vi "Increment Waveform.vi"(8 "error in (no error)":errorcluster, 11 "Model in":refnum<class "Model.lvclass">) -> (0 "error out":errorcluster, 3 "Model out":refnum<class "Model.lvclass">)   [LabVIEW 2016]
uses:
  Model.lvclass
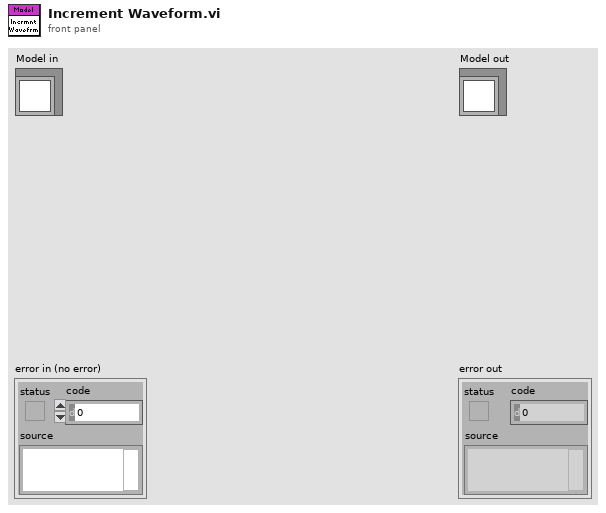
[diagram p1: front panel]
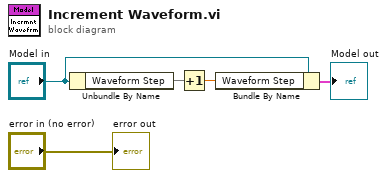
[diagram p0: block diagram]
diagram:
  n1 = Unbundle By Name("Model in") -> ("Waveform Step"=w4)
  n2 = Increment(x=w4) -> (x+1=w1:dbl)
  n3 = Bundle By Name(cluster="Model in", "Waveform Step"=w1) -> (→"Model out":cluster{})
  "error out" <- "error in (no error)"
